vi "Test01SN.vi"(8 "errin":errorcluster, 11 "String":string) -> (0 "errout":errorcluster)   [LabVIEW 2020]
uses:
  VarGLO/Global Limite de test.vi
  <vilib>/regexp/Match Regular Expression.xnode
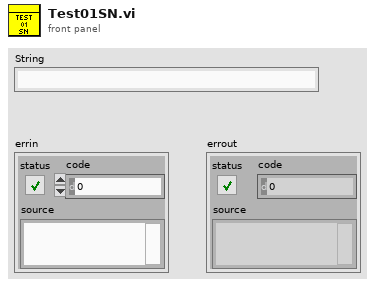
[diagram p1: front panel]
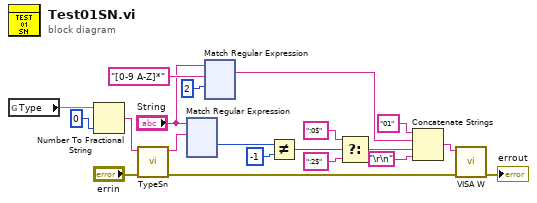
[diagram p0: block diagram]
diagram:
  n1 = global read "Global Limite de test.vi" "Type"() -> (w4:dbl)
  n2 = Number To Fractional String ("Nombre en chaîne fractionnaire")(number=w4, precision (6)=i16 0 ("précision (6)")) -> (F-format string=w12:string)  [unwired: 2 in]
  n3 = call "TypeSn.vi"("errin"="errin", "ModuleType"=w12) -> ("error out"=w3:errorcluster, "root sn"=w15:string)  [unwired: 8 in]
  n4 = xnode "Match Regular Expression"("chaîne en entrée"="String", "expression régulière"=w15) -> ("offset après correspondance"=w16:i32)  [unwired: 4 in, 4 out]
  n5 = xnode "Match Regular Expression"("chaîne en entrée"="String", "expression régulière"="[0-9 A-Z]*", "offset (0)"=2) -> ("toute l'expression"=w10:string)  [unwired: 3 in, 4 out]
  n6 = Not Equal? ("Différents ?")(x=w16, y=-1) -> (x != y?=w18:bool)
  n7 = Select ("Sélectionner")(t=":0$" ("chaîne"), s=w18, f=":2$" ("cas faux")) -> (s? t:f=w13:string)
  n8 = Concatenate Strings("01" ("chaîne"), w10, w13, "\r\n") -> (w1:string)
  n9 = call "VISA W.vi"("errin"=w3, "Chaîne"=w1) -> ("errout"=→"errout":errorcluster)  [unwired: 9 in]
